vi "PM5000_SagSwell_Alarmas.vi"(8 "error in":errorcluster, 11 "Network Path":string="172.22.26.202") -> (0 "error out":errorcluster, 2 "PQ_Alarmas":bool[](array[boolean]), 3 "Network Path out":string="192.168.169.1")   [LabVIEW 2018]
doc: "Lee la tabla de memoria RealTime_VIF_Power del equipo PowerMonitor 5000, ademas filtra y ordena las variables de interez de la tabla de memoria.\n\nLee las siguientes variables de la tabla RealTime_VIF_Power:\n\n*V1_V2_Volts\n*V2_V3_Volts\n*V3_V1_Volts\n*I1_Amps\n*I2_Amps\n*I3_Amps\n*Frequency_Hz\n*Total_kW\n*Total_kVAR\n*Total_kVA\n*Total_True_PF\n*Total_Disp_PF"
uses:
  <vilib>/ethernetip/ethernetip.llb/EthernetIP SLC500 Read Integer.vi
  <vilib>/ethernetip/ethernetip.lvlib
panel:
  # "Sag_Indication_Detected"
  # "Swell_Indication_Detected"
  # "Transient_Indication"
  # "200mS_Sag_Swell_Status_Flag"
  # "3s_Sag_Swell_Status_Flag"
  # "10m_Sag_Swell_Status_Flag"
  # "2h_Sag_Swell_Status_Flag"
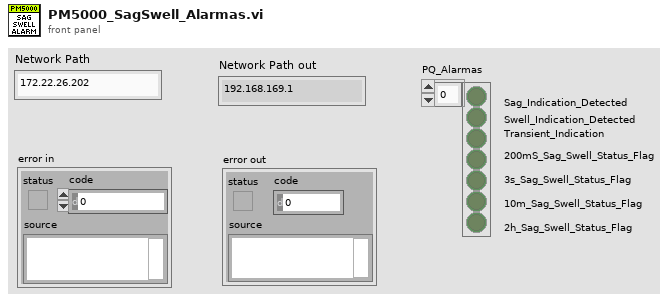
[diagram p1: front panel]
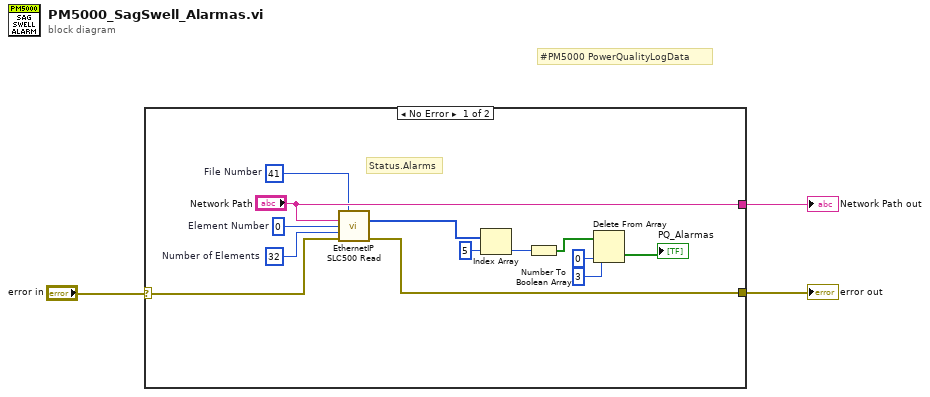
[diagram p0: block diagram]
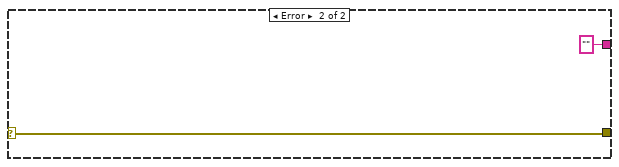
[diagram p2: hidden frame]
diagram:
  # "#PM5000 PowerQualityLogData"
  n1 = case shown="No Error" "error in" {
    selector: "error in" -> [w11 w18]
    tunnel: [w16 w18] -> w3
    tunnel: ["Network Path" "" ("Network Path")] -> w2
    frame No Error {
      w12 = u32 32  # Number of Elements
      w14 = u16 41  # File Number
      w13 = u16 0  # Element Number
      # "Status.Alarms"
      n2 = call-poly <vilib>:"EthernetIP SLC500 Read.vi"("File Number"=w14, "Network Path"="Network Path", "Element Number"=w13, "Number of Elements"=w12, "error in"=w11) -> ("Data"=w10:i16[], "error out"=w16:errorcluster)  [unwired: 8 in, 1 out]
      n3 = Index Array(array=w10, index=5) -> (element=w9:i16)
      n4 = Number To Boolean Array(number=w9) -> (Boolean array=w7:bool[])
      n5 = Delete From Array(array=w7, length=3, index=0) -> (deleted portion=→"PQ_Alarmas":bool[])  [unwired: 1 out]
    }
    frame Error {
    }
  }
  "error out" <- w3
  "Network Path out" <- w2
